vi "Measurement.Free.GetPublicEventsRegistration.vi"(8 "error in (no error)":errorcluster, 11 "Measurement.Free":refnum<class "Measurement.Free.lvclass">) -> (0 "error out":errorcluster, 2 "Measurement.Free Public Events":refnum<event-registration>, 3 "Measurement.Free out":refnum<class "Measurement.Free.lvclass">)   [LabVIEW 2017, in "Measurement.Free.lvclass"]
doc: "---------------------------------------------------------------\nJKI State Machine Objects™\nhttp://jki.net/state-machine-objects/\nCopyright (C) 2005-2015, JKI <info@jki.net>\nALL RIGHTS RESERVEDJKI State Machine Objects (SMO) 1.0.0.5\nJKI - JKI\nCopyright (c) 2016, JKI"
uses:
  Measurement.Free.lvclass
  Typedefs/PublicEvents--Cluster.ctl
  Typedefs/DataChanged--EventData--Cluster.ctl
  Typedefs/Data.ctl
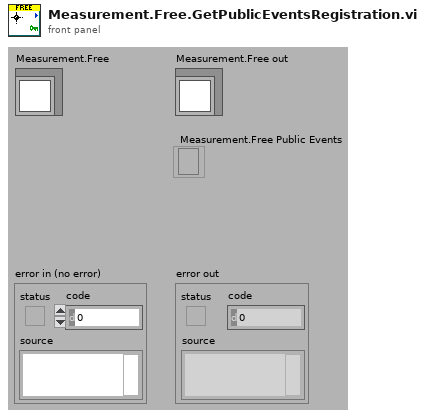
[diagram p1: front panel]
types:
  T1 = typedef "Measurement.Free.lvclass/PublicEvents--Cluster.ctl" = cluster{"Data Changed":refnum<user-event>}
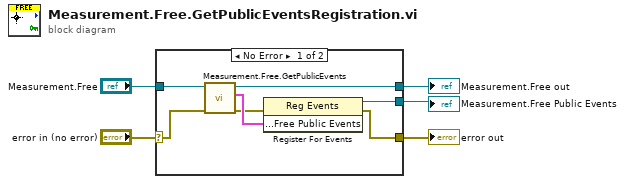
[diagram p0: block diagram]
diagram:
  n1 = case shown="No Error" "error in (no error)" {
    selector: "error in (no error)" -> [w11 w13]
    tunnel: "Measurement.Free" -> [w12 w14]
    tunnel: [w6 w13] -> w4
    tunnel: [w7 w14] -> w3
    tunnel: [w8 _] -> w1
    frame No Error {
      n2 = call "Measurement.Free.GetPublicEvents.vi"("error in (no error)"=w11, "Measurement.Free"=w12) -> ("error out"=w9:errorcluster, "Measurement.Free Public Events"=w10:T1, "Measurement.Free out"=w7:refnum<class "Measurement.Free.lvclass">)  [unwired: 7 in]
      n3 = register-events(error in=w9, w10) -> (reference out=w8:refnum<event-registration>, error out=w6:errorcluster)  [unwired: 1 in]
    }
    frame Error {
    }
  }
  "error out" <- w4
  "Measurement.Free out" <- w3
  "Measurement.Free Public Events" <- w1
